vi "Local Bus Test.vi"() -> ()   [LabVIEW 2021]
uses:
  Source/Omni-Bus/Omni_Bus.lvclass
  Source/Omni-Bus/Support/Broad Types.ctl
  Source/Local Bus/Local Bus.lvclass
  C:/Users/Tim/Documents/GitHub/Omni-Bus/Source/Omni-Bus/Bus Access/Bus_Access.lvclass
  <vilib>/Utility/Data Type/Type Definitions/Data Type.ctl
  Source/Local Bus/Local Bus.lvclass/Local Bus.ctl
  Source/Omni-Bus/Write/Write CSGL.vi
  Source/Local Bus/Properties/Write Tag List.vi
  <vilib>/TSA/Abstract Data Classes/Abs_Types/Complex Single Float/Abs_Complex Single Float.lvclass
  <vilib>/TSA/Abstract Data Classes/Abs_Types/U8 Integer/Abs_U8 Integer.lvclass
  <vilib>/Utility/Data Type/NI_Data Type.lvlib
  Source/Omni-Bus/Read/Read DBL.vi
panel:
  out "error out 3":errorcluster
  out "error out 2":errorcluster
  in  "Numeric 2":csg
  in  "Tag 2":string
  in  "stop":bool
  out "Numeric":dbl format="%.2f"
  in  "Tag":string
  out "error out":errorcluster
  out "Tags":string[](array[string])
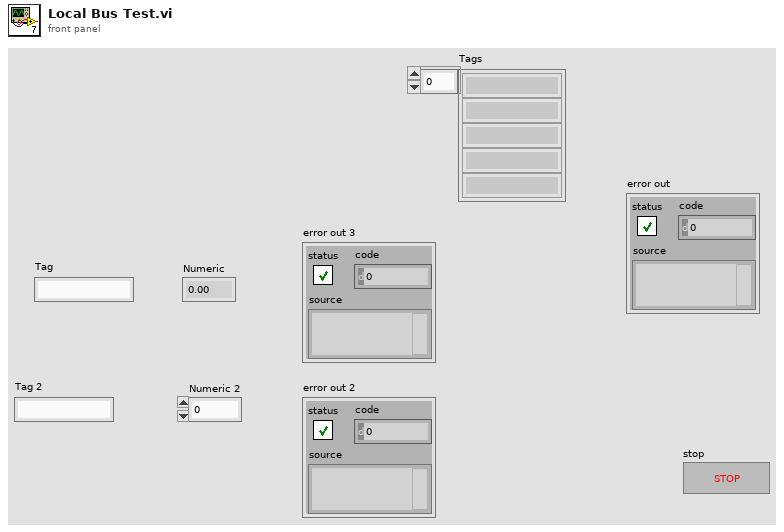
[diagram p1: front panel]
types:
  T1 = typedef "NI_Data Type.lvlib/Data Type.ctl" = enum8{"Invalid Type", "Void", "I8", "I16", "I32", "I64", "U8", "U16", "U32", "U64", "Single Float", "Double Float", "Extended Float", "Single Complex", "Double Complex", "Extended Complex", "Enum U8", "Enum U16", "Enum U32", "Enum U64", "Single Float With Unit", "Double Float With Unit", "Extended Float With Unit", "Single Complex with Unit", "Double Complex with Unit", "Extended Complex with Unit", "Boolean", "String", "Path", "Picture", "Tag", "Array", "Cluster", "Variant", "LV Variant", "Waveform", "Timestamp", "Digital Waveform", "Digital Data", "ExpressData", "Refnum", "External Data", "VI", "Poly VI", "LabVIEW Class Instance", "Fixed Point", "Set Collection", "Map Collection"}
  T2 = typedef "Omni_Bus.lvclass/Broad Types.ctl" = enum16{"All Tags", "NI Specific Type", "Boolean", "String", "Numeric", "Float", "Integer", "Collection", "All Value Types", "Non Value Types"}
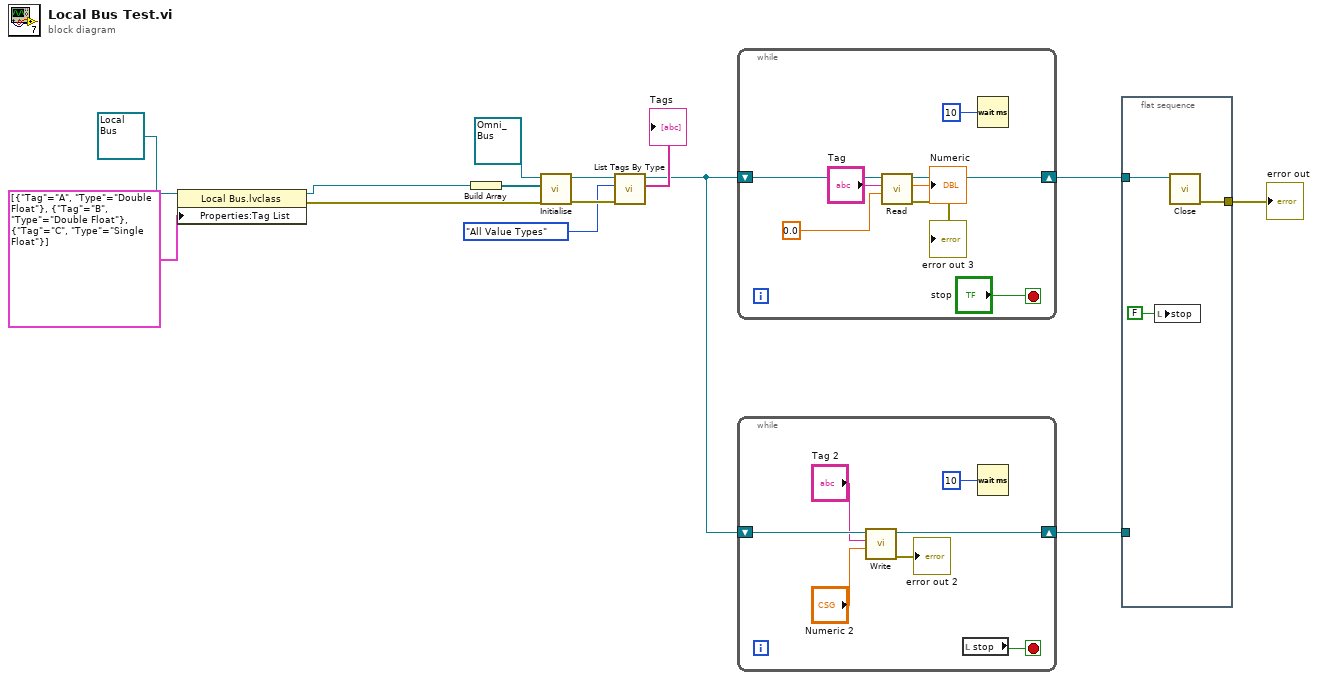
[diagram p0: block diagram]
diagram:
  n1 = property class="Local Bus.lvclass"(reference=refnum<class "Local Bus.lvclass"> refnum ("Local Bus.lvclass"), "Properties:Tag List"=cluster{"Tag":string, "Type":T1}[] [{"Tag"="A", "Type"=enum."Double Float"}, {"Tag"="B", "Type"=enum."Double Float"}, {"Tag"="C", "Type"=enum."Single Float"}] ("Tag List")) -> (reference out=w7:refnum<class "Local Bus.lvclass">, error out=w6:errorcluster)  [unwired: 1 in]
  n2 = Build Array(w7) -> (w13:refnum<class "Local Bus.lvclass">[])
  n3 = call-dynamic "Initialise.vi"("error in (no error)"=w6, "Bus Access"=w13, "Var Bus in"=refnum<class "Omni_Bus.lvclass"> refnum) -> ("error out"=w11:errorcluster, "Var Bus out"=w12:refnum<class "Omni_Bus.lvclass">)  [unwired: 7 in]
  n4 = call-dynamic "List Tags By Type.vi"("error in (no error)"=w11, "Broad Types"=Broad_Types."All Value Types", "Var Bus in"=w12) -> ("Tags"=→"Tags":string[], "Var Bus out"=w2:refnum<class "Omni_Bus.lvclass">)  [unwired: 5 in, 2 out]
  n5 = while {
    shift-right: [w21] -> w3
    shift-left: w2 -> [w22]
    stop <- "stop" stop-if-true
    n6 = call-poly "Read.vi"("Type"=0.0 ("Poly Type"), "Tag"="Tag", "Var Bus in"=w22) -> ("error out"=→"error out 3":errorcluster, "Numeric"=→"Numeric":dbl, "Var Bus out"=w21:refnum<class "Omni_Bus.lvclass">)  [unwired: 6 in]
    n7 = Wait (ms)(milliseconds to wait=u32 10) -> ()  [unwired: 1 out]
  }
  n8 = while {
    shift-right: [w28] -> w1
    shift-left: w2 -> [w29]
    stop <- w25 stop-if-true
    n9 = call-poly "Write.vi"("Numeric"="Numeric 2", "Tag"="Tag 2", "Omni_Bus in"=w29) -> ("error out"=→"error out 2":errorcluster, "Omni_Bus out"=w28:refnum<class "Omni_Bus.lvclass">)  [unwired: 7 in]
    n10 = local read "stop"() -> (w25:bool)
    n11 = Wait (ms)(milliseconds to wait=u32 10) -> ()  [unwired: 1 out]
  }
  n12 = flat-sequence {
    tunnel: [w32] -> w8
    tunnel: w3 -> [w31]
    tunnel: w1 -> [_]
    frame #0 {
      n13 = local write "stop"(FALSE ("stop")) -> ()
      n14 = call-dynamic "Close.vi"("Data in"=w31) -> ("error out"=w32:errorcluster)  [unwired: 9 in, 1 out]
    }
  }
  "error out" <- w8
